vi "Autonomous Independent.vi"   [LabVIEW 2016]
doc: "This VI is called when autonomous begins, and will automatically be terminated when autonomous ends. You can carry out timed or sensor driven robot movement independently without needing to return to the caller."
uses:
  <vilib>/Rock Robotics/WPI/SafetyOutput/WPI_SafetyOutputConfigMenu.ctl
  <vilib>/Rock Robotics/WPI/Utilities/WPI_GetSetVariantRefNum.vi
  <vilib>/Rock Robotics/WPI/RobotDrive/WPI_RobotDriveArcadeDrive_Standard(NoSaturation).vi
panel:
  # "Be sure to right-click and choose Data Operations>>Make Current Value default if you want to save the array values with the VI"
types:
  T1 = typedef "WPI_SafetyOutputConfigMenu.ctl" = enum16{"Enable", "Disable"}
  T2 = typedef "WPI_JoystickDevRef.ctl" = cluster{"Device":T3}
  T3 = typedef "WPI_JoystickDeviceEnum.ctl" = enum16{"USB 0", "USB 1", "USB 2", "USB 3", "USB 4", "USB 5"}
  T4 = typedef "WPI_RobotDriveDevRef.ctl" = cluster{"DevStatus":errorcluster, "Motors[]":T5[], "Square Inputs":bool, "Max Output":dbl}
  T5 = typedef "WPI_MotorControlDeviceRef.ctl" = cluster{"DeviceStatus":errorcluster, "Type":T6, "PWM":cluster{"PWM Channel":T7, "DeadBand":T8}, "CAN":cluster{"Device Number":u8, "SetOutput VI Ref":variant, "GetOutput VI Ref":variant, "Enable VI Ref":variant, "Disable VI Ref":variant, "Data":variant}, "Invert":bool}
  T6 = typedef "WPI_MotorControlType.ctl" = enum16{"PWM", "CAN"}
  T7 = typedef "FPGA_DIOPWMChannel.ctl" = enum8{"PWM 0", "PWM 1", "PWM 2", "PWM 3", "PWM 4", "PWM 5", "PWM 6", "PWM 7", "PWM 8", "PWM 9", "PWM MXP 0", "PWM MXP 1", "PWM MXP 2", "PWM MXP 3", "PWM MXP 4", "PWM MXP 5", "PWM MXP 6", "PWM MXP 7", "PWM MXP 8", "PWM MXP 9", "Invalid"}
  T8 = typedef "WPI_PWMDeadband.ctl" = cluster{"Name":string, "maxPositivePwm":i32, "minPositivePwm":i32, "centerPwm":i32, "maxNegativePwm":i32, "minNegativePwm":i32, "angularRange":u16}
  T9 = cluster{"Buttons[0]":bool, "Buttons[1]":bool, "Buttons[2]":bool, "Buttons[3]":bool, "Buttons[4]":bool, "Buttons[5]":bool, "Buttons[6]":bool, "Buttons[7]":bool, "Buttons[8]":bool}
  T10 = cluster{"Yaw":dbl, "Roll":dbl, "Pitch":dbl, "Heading":dbl, "Fused Heading":dbl}
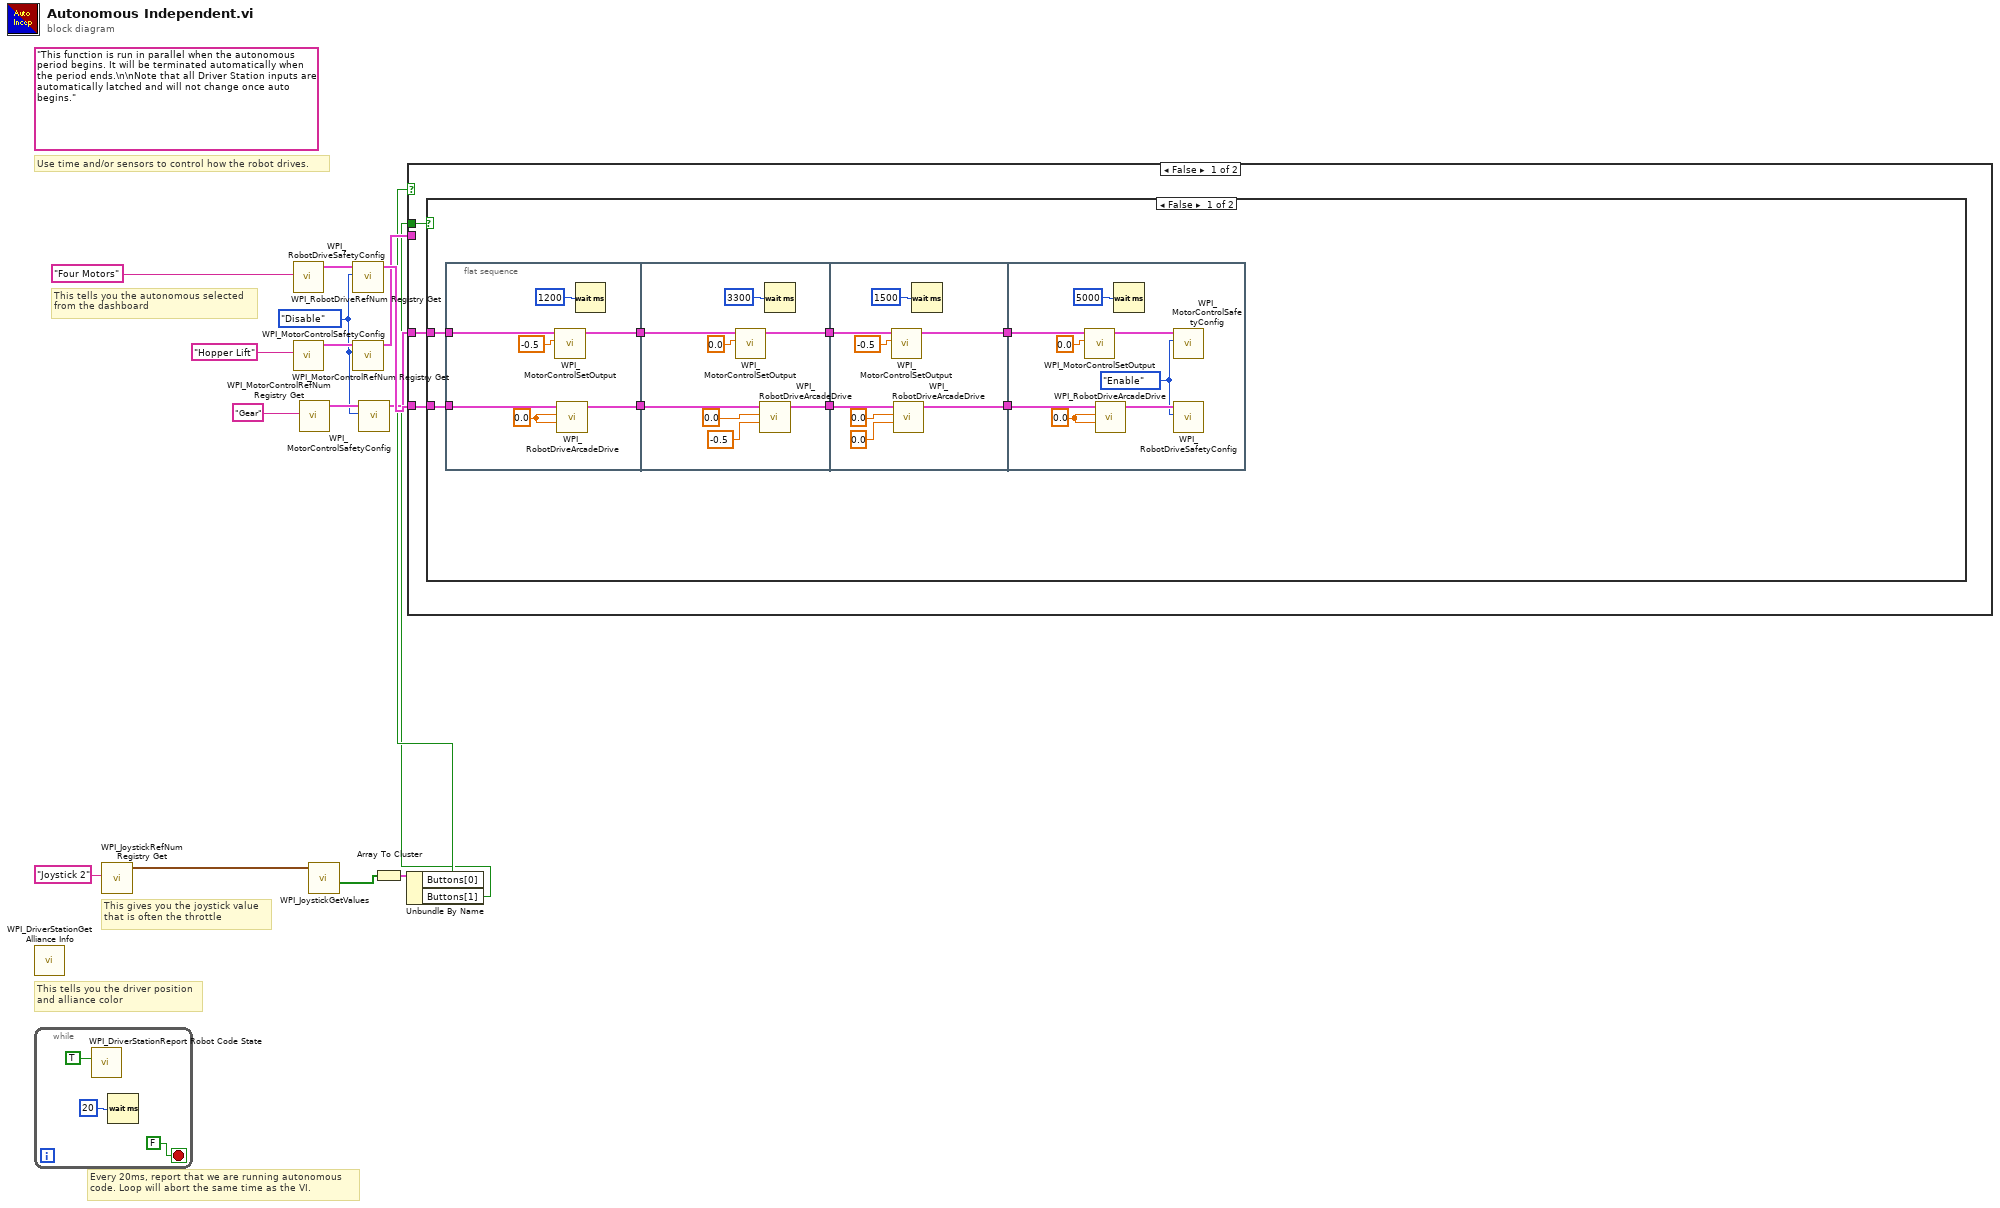
[diagram p0: block diagram]
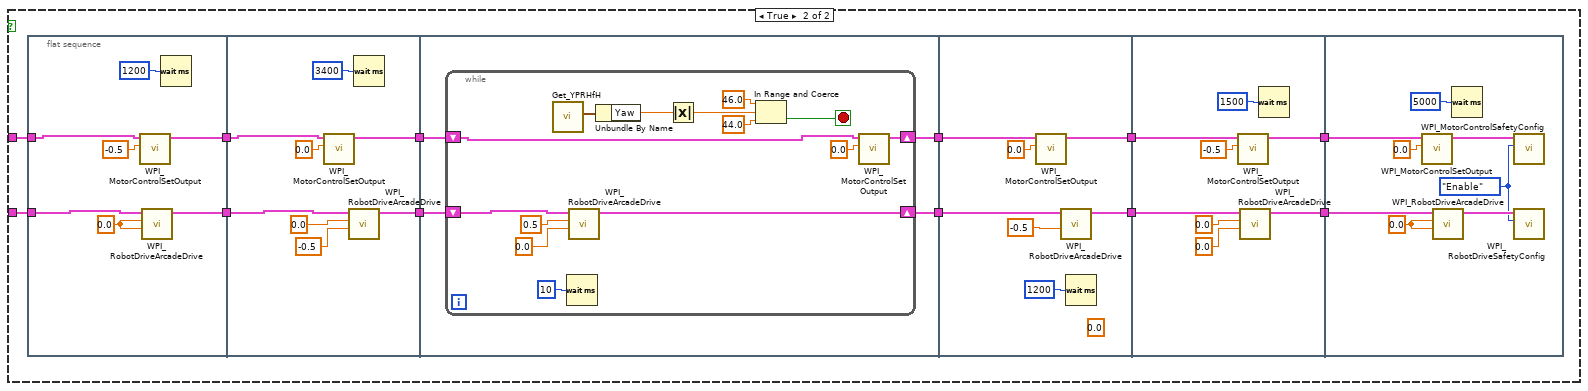
[diagram p2: hidden frame]
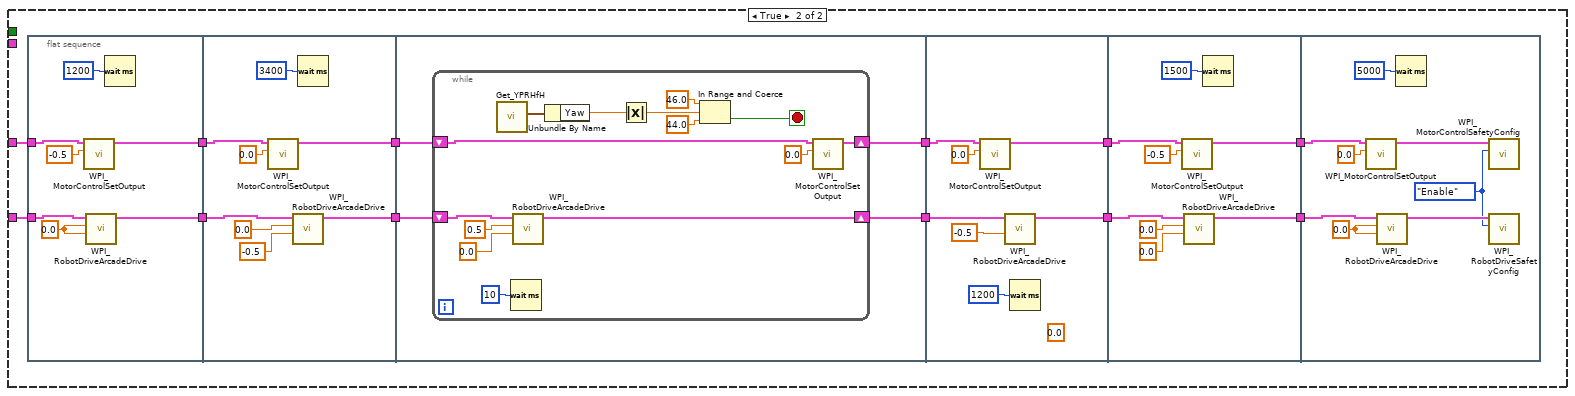
[diagram p3: hidden frame]
diagram:
  w6 = WPI_SafetyOutputConfigMenu."Disable" ("mode")
  (unwired) "This function is run in parallel when the autonomous period begins. It will be terminated automatically when the period ends.\n\nNote that all Driver Station inputs are automatically latched and will not change once auto begins."
  # "This tells you the autonomous selected\nfrom the dashboard"
  # "Every 20ms, report that we are running autonomous\ncode. Loop will abort the same time as the VI."
  # "This gives you the joystick value\nthat is often the throttle"
  # "Use time and/or sensors to control how the robot drives."
  # "This tells you the driver position\nand alliance color"
  n1 = call <vilib>:"WPI_DriverStationGet Alliance Info.vi"() -> ()  [unwired: 12 out]
  n2 = while {
    stop <- FALSE stop-if-true
    n3 = call <vilib>:"WPI_DriverStationReport Robot Code State.vi"("Autonomous"=TRUE) -> ()  [unwired: 10 in, 1 out]
    n4 = Wait (ms)(milliseconds to wait=u32 20) -> ()  [unwired: 1 out]
  }
  n5 = call <vilib>:"WPI_JoystickRefNum Registry Get.vi"("refnum name"="Joystick 2") -> ("JoystickDevRef"=w15:T2)  [unwired: 1 in, 9 out]
  n6 = call <vilib>:"WPI_RobotDriveRefNum Registry Get.vi"("refnum name"="Four Motors") -> ("RobotDriveDevRef"=w13:T4)  [unwired: 1 in, 9 out]
  n7 = call <vilib>:"WPI_MotorControlRefNum Registry Get.vi"("refnum name"="Hopper Lift") -> ("MotorControlDevRef"=w11:T5)  [unwired: 9 in, 1 out]
  n8 = call <vilib>:"WPI_MotorControlRefNum Registry Get.vi"("refnum name"="Gear") -> ("MotorControlDevRef"=w7:T5)  [unwired: 9 in, 1 out]
  n9 = call <vilib>:"WPI_JoystickGetValues.vi"("JoystickDevRef"=w15) -> ("Buttons"=w4:bool[])  [unwired: 6 in, 4 out]
  n10 = call <vilib>:"WPI_RobotDriveSafetyConfig.vi"("mode"=w6, "RobotDriveDevRef"=w13) -> ("RobotDriveDevRef"=w12:T4)  [unwired: 8 in, 1 out]
  n11 = call <vilib>:"WPI_MotorControlSafetyConfig.vi"("mode"=w6, "MotorControlDevRef"=w11) -> ("MotorControlDevRef"=w9:T5)  [unwired: 8 in, 1 out]
  n12 = call <vilib>:"WPI_MotorControlSafetyConfig.vi"("mode"=w6, "MotorControlDevRef"=w7) -> ("MotorControlDevRef"=w5:T5)  [unwired: 8 in, 1 out]
  n13 = Array To Cluster(array=w4) -> (cluster=w1:T9)
  n14 = Unbundle By Name(w1) -> ("Buttons[0]"=w3:bool, "Buttons[1]"=w2:bool)
  n15 = case shown="False" w3 {
    tunnel: w12 -> [w22 w130]
    tunnel: w9 -> [_ _]
    tunnel: w5 -> [w21 w131]
    tunnel: w2 -> [w20 _]
    frame False {
      n16 = case shown="False" w20 {
        tunnel: w22 -> [w28 w69]
        tunnel: w21 -> [w27 w68]
        frame False {
          n17 = flat-sequence {
            tunnel: w28 -> [w37]
            tunnel: [w36] -> w30
            tunnel: w27 -> [w34]
            tunnel: [w33] -> w29
            tunnel: w30 -> [w45]
            tunnel: [w44] -> w26
            tunnel: [w43] -> w24
            tunnel: w29 -> [w42]
            tunnel: w26 -> [w49]
            tunnel: [w48] -> w25
            tunnel: w24 -> [w47]
            tunnel: [w46] -> w23
            tunnel: w25 -> [w61]
            tunnel: w23 -> [w58]
            frame #0 {
              w35 = 0.0 ("X axis value")
              n18 = call <vilib>:"WPI_MotorControlSetOutput.vi"("Output"=-0.5, "MotorControlDevRef"=w34) -> ("MotorControlDevRef"=w33:T5)  [unwired: 7 in, 2 out]
              n19 = call-poly <vilib>:"WPI_RobotDriveArcadeDrive.vi"("Y axis value"=w35, "X axis value"=w35, "RobotDriveDevRef"=w37) -> ("RobotDriveDevRef"=w36:T4)  [unwired: 6 in, 2 out]
              n20 = Wait (ms)(milliseconds to wait=u32 1200) -> ()  [unwired: 1 out]
            }
            frame #1 {
              n21 = call <vilib>:"WPI_MotorControlSetOutput.vi"("Output"=0.0, "MotorControlDevRef"=w42) -> ("MotorControlDevRef"=w43:T5)  [unwired: 7 in, 2 out]
              n22 = call-poly <vilib>:"WPI_RobotDriveArcadeDrive.vi"("Y axis value"=-0.5, "X axis value"=0.0, "RobotDriveDevRef"=w45) -> ("RobotDriveDevRef"=w44:T4)  [unwired: 6 in, 2 out]
              n23 = Wait (ms)(milliseconds to wait=u32 3300) -> ()  [unwired: 1 out]
            }
            frame #2 {
              n24 = call <vilib>:"WPI_MotorControlSetOutput.vi"("Output"=-0.5, "MotorControlDevRef"=w47) -> ("MotorControlDevRef"=w46:T5)  [unwired: 7 in, 2 out]
              n25 = call-poly <vilib>:"WPI_RobotDriveArcadeDrive.vi"("Y axis value"=0.0, "X axis value"=0.0, "RobotDriveDevRef"=w49) -> ("RobotDriveDevRef"=w48:T4)  [unwired: 6 in, 2 out]
              n26 = Wait (ms)(milliseconds to wait=u32 1500) -> ()  [unwired: 1 out]
            }
            frame #3 {
              w59 = 0.0 ("Y axis value")
              w56 = WPI_SafetyOutputConfigMenu."Enable" ("mode")
              n27 = call <vilib>:"WPI_MotorControlSetOutput.vi"("Output"=0.0, "MotorControlDevRef"=w58) -> ("MotorControlDevRef"=w57:T5)  [unwired: 7 in, 2 out]
              n28 = call-poly <vilib>:"WPI_RobotDriveArcadeDrive.vi"("Y axis value"=w59, "X axis value"=w59, "RobotDriveDevRef"=w61) -> ("RobotDriveDevRef"=w60:T4)  [unwired: 6 in, 2 out]
              n29 = Wait (ms)(milliseconds to wait=u32 5000) -> ()  [unwired: 1 out]
              n30 = call <vilib>:"WPI_MotorControlSafetyConfig.vi"("mode"=w56, "MotorControlDevRef"=w57) -> ()  [unwired: 8 in, 2 out]
              n31 = call <vilib>:"WPI_RobotDriveSafetyConfig.vi"("mode"=w56, "RobotDriveDevRef"=w60) -> ()  [unwired: 8 in, 2 out]
            }
          }
        }
        frame True {
          n32 = flat-sequence {
            tunnel: w69 -> [w80]
            tunnel: [w79] -> w73
            tunnel: w68 -> [w77]
            tunnel: [w76] -> w72
            tunnel: w73 -> [w88]
            tunnel: [w87] -> w67
            tunnel: [w86] -> w66
            tunnel: w72 -> [w85]
            tunnel: w67 -> [w90]
            tunnel: w66 -> [w91]
            tunnel: [w89] -> w64
            tunnel: [w92] -> w63
            tunnel: [w110] -> w65
            tunnel: w64 -> [w108]
            tunnel: w63 -> [w111]
            tunnel: [w107] -> w62
            tunnel: [w117] -> w71
            tunnel: w65 -> [w116]
            tunnel: [w115] -> w70
            tunnel: w62 -> [w114]
            tunnel: w71 -> [w129]
            tunnel: w70 -> [w126]
            frame #0 {
              w78 = 0.0 ("X axis value")
              n33 = call <vilib>:"WPI_MotorControlSetOutput.vi"("Output"=-0.5, "MotorControlDevRef"=w77) -> ("MotorControlDevRef"=w76:T5)  [unwired: 7 in, 2 out]
              n34 = call-poly <vilib>:"WPI_RobotDriveArcadeDrive.vi"("Y axis value"=w78, "X axis value"=w78, "RobotDriveDevRef"=w80) -> ("RobotDriveDevRef"=w79:T4)  [unwired: 6 in, 2 out]
              n35 = Wait (ms)(milliseconds to wait=u32 1200) -> ()  [unwired: 1 out]
            }
            frame #1 {
              n36 = call <vilib>:"WPI_MotorControlSetOutput.vi"("Output"=0.0, "MotorControlDevRef"=w85) -> ("MotorControlDevRef"=w86:T5)  [unwired: 7 in, 2 out]
              n37 = call-poly <vilib>:"WPI_RobotDriveArcadeDrive.vi"("Y axis value"=-0.5, "X axis value"=0.0, "RobotDriveDevRef"=w88) -> ("RobotDriveDevRef"=w87:T4)  [unwired: 6 in, 2 out]
              n38 = Wait (ms)(milliseconds to wait=u32 3400) -> ()  [unwired: 1 out]
            }
            frame #2 {
              n39 = while {
                shift-right: [w101] -> w92
                shift-left: w91 -> [w104]
                shift-right: [w102] -> w89
                shift-left: w90 -> [w103]
                stop <- w99 stop-if-true
                n40 = call <vilib>:"Get_YPRHfH.vi"() -> ("YRPHfH"=w96:T10)  [unwired: 11 in]
                n41 = Wait (ms)(milliseconds to wait=u32 10) -> ()  [unwired: 1 out]
                n42 = call-poly <vilib>:"WPI_RobotDriveArcadeDrive.vi"("Y axis value"=0.0 ("X axis value"), "X axis value"=0.5 ("Y axis value"), "RobotDriveDevRef"=w103) -> ("RobotDriveDevRef"=w102:T4)  [unwired: 6 in, 2 out]
                n43 = Unbundle By Name(w96) -> ("Yaw"=w95:dbl)
                n44 = Absolute Value(x=w95) -> (abs(x)=w94:dbl)
                n45 = In Range and Coerce(upper limit=46.0, x=w94, lower limit=44.0) -> (In Range?=w99:bool)  [unwired: 1 out]
                n46 = call <vilib>:"WPI_MotorControlSetOutput.vi"("Output"=0.0, "MotorControlDevRef"=w104) -> ("MotorControlDevRef"=w101:T5)  [unwired: 7 in, 2 out]
              }
            }
            frame #3 {
              (unwired) 0.0 ("X axis value")
              n47 = call <vilib>:"WPI_MotorControlSetOutput.vi"("Output"=0.0, "MotorControlDevRef"=w111) -> ("MotorControlDevRef"=w110:T5)  [unwired: 7 in, 2 out]
              n48 = call-poly <vilib>:"WPI_RobotDriveArcadeDrive.vi"("Y axis value"=-0.5, "RobotDriveDevRef"=w108) -> ("RobotDriveDevRef"=w107:T4)  [unwired: 7 in, 2 out]
              n49 = Wait (ms)(milliseconds to wait=u32 1200) -> ()  [unwired: 1 out]
            }
            frame #4 {
              n50 = call <vilib>:"WPI_MotorControlSetOutput.vi"("Output"=-0.5, "MotorControlDevRef"=w116) -> ("MotorControlDevRef"=w115:T5)  [unwired: 7 in, 2 out]
              n51 = call-poly <vilib>:"WPI_RobotDriveArcadeDrive.vi"("Y axis value"=0.0, "X axis value"=0.0, "RobotDriveDevRef"=w114) -> ("RobotDriveDevRef"=w117:T4)  [unwired: 6 in, 2 out]
              n52 = Wait (ms)(milliseconds to wait=u32 1500) -> ()  [unwired: 1 out]
            }
            frame #5 {
              w127 = 0.0 ("Y axis value")
              w124 = WPI_SafetyOutputConfigMenu."Enable" ("mode")
              n53 = call <vilib>:"WPI_MotorControlSetOutput.vi"("Output"=0.0, "MotorControlDevRef"=w126) -> ("MotorControlDevRef"=w125:T5)  [unwired: 7 in, 2 out]
              n54 = call-poly <vilib>:"WPI_RobotDriveArcadeDrive.vi"("Y axis value"=w127, "X axis value"=w127, "RobotDriveDevRef"=w129) -> ("RobotDriveDevRef"=w128:T4)  [unwired: 6 in, 2 out]
              n55 = Wait (ms)(milliseconds to wait=u32 5000) -> ()  [unwired: 1 out]
              n56 = call <vilib>:"WPI_MotorControlSafetyConfig.vi"("mode"=w124, "MotorControlDevRef"=w125) -> ()  [unwired: 8 in, 2 out]
              n57 = call <vilib>:"WPI_RobotDriveSafetyConfig.vi"("mode"=w124, "RobotDriveDevRef"=w128) -> ()  [unwired: 8 in, 2 out]
            }
          }
        }
      }
    }
    frame True {
      n58 = flat-sequence {
        tunnel: w130 -> [w148]
        tunnel: [w147] -> w141
        tunnel: w131 -> [w145]
        tunnel: [w144] -> w140
        tunnel: w141 -> [w156]
        tunnel: [w155] -> w139
        tunnel: [w154] -> w138
        tunnel: w140 -> [w153]
        tunnel: w139 -> [w159]
        tunnel: w138 -> [w160]
        tunnel: [w158] -> w137
        tunnel: [w157] -> w136
        tunnel: [w178] -> w135
        tunnel: w137 -> [w176]
        tunnel: w136 -> [w179]
        tunnel: [w175] -> w134
        tunnel: [w185] -> w133
        tunnel: w135 -> [w184]
        tunnel: [w183] -> w132
        tunnel: w134 -> [w182]
        tunnel: w133 -> [w197]
        tunnel: w132 -> [w194]
        frame #0 {
          w146 = 0.0 ("X axis value")
          n59 = call <vilib>:"WPI_MotorControlSetOutput.vi"("Output"=-0.5, "MotorControlDevRef"=w145) -> ("MotorControlDevRef"=w144:T5)  [unwired: 7 in, 2 out]
          n60 = call-poly <vilib>:"WPI_RobotDriveArcadeDrive.vi"("Y axis value"=w146, "X axis value"=w146, "RobotDriveDevRef"=w148) -> ("RobotDriveDevRef"=w147:T4)  [unwired: 6 in, 2 out]
          n61 = Wait (ms)(milliseconds to wait=u32 1200) -> ()  [unwired: 1 out]
        }
        frame #1 {
          n62 = call <vilib>:"WPI_MotorControlSetOutput.vi"("Output"=0.0, "MotorControlDevRef"=w153) -> ("MotorControlDevRef"=w154:T5)  [unwired: 7 in, 2 out]
          n63 = call-poly <vilib>:"WPI_RobotDriveArcadeDrive.vi"("Y axis value"=-0.5, "X axis value"=0.0, "RobotDriveDevRef"=w156) -> ("RobotDriveDevRef"=w155:T4)  [unwired: 6 in, 2 out]
          n64 = Wait (ms)(milliseconds to wait=u32 3400) -> ()  [unwired: 1 out]
        }
        frame #2 {
          n65 = while {
            shift-right: [w169] -> w157
            shift-left: w160 -> [w172]
            shift-right: [w170] -> w158
            shift-left: w159 -> [w171]
            stop <- w167 stop-if-true
            n66 = call <vilib>:"Get_YPRHfH.vi"() -> ("YRPHfH"=w164:T10)  [unwired: 11 in]
            n67 = Wait (ms)(milliseconds to wait=u32 10) -> ()  [unwired: 1 out]
            n68 = call-poly <vilib>:"WPI_RobotDriveArcadeDrive.vi"("Y axis value"=0.0 ("X axis value"), "X axis value"=0.5 ("Y axis value"), "RobotDriveDevRef"=w171) -> ("RobotDriveDevRef"=w170:T4)  [unwired: 6 in, 2 out]
            n69 = Unbundle By Name(w164) -> ("Yaw"=w163:dbl)
            n70 = Absolute Value(x=w163) -> (abs(x)=w162:dbl)
            n71 = In Range and Coerce(upper limit=46.0, x=w162, lower limit=44.0) -> (In Range?=w167:bool)  [unwired: 1 out]
            n72 = call <vilib>:"WPI_MotorControlSetOutput.vi"("Output"=0.0, "MotorControlDevRef"=w172) -> ("MotorControlDevRef"=w169:T5)  [unwired: 7 in, 2 out]
          }
        }
        frame #3 {
          (unwired) 0.0 ("X axis value")
          n73 = call <vilib>:"WPI_MotorControlSetOutput.vi"("Output"=0.0, "MotorControlDevRef"=w179) -> ("MotorControlDevRef"=w178:T5)  [unwired: 7 in, 2 out]
          n74 = call-poly <vilib>:"WPI_RobotDriveArcadeDrive.vi"("Y axis value"=-0.5, "RobotDriveDevRef"=w176) -> ("RobotDriveDevRef"=w175:T4)  [unwired: 7 in, 2 out]
          n75 = Wait (ms)(milliseconds to wait=u32 1200) -> ()  [unwired: 1 out]
        }
        frame #4 {
          n76 = call <vilib>:"WPI_MotorControlSetOutput.vi"("Output"=-0.5, "MotorControlDevRef"=w184) -> ("MotorControlDevRef"=w183:T5)  [unwired: 7 in, 2 out]
          n77 = call-poly <vilib>:"WPI_RobotDriveArcadeDrive.vi"("Y axis value"=0.0, "X axis value"=0.0, "RobotDriveDevRef"=w182) -> ("RobotDriveDevRef"=w185:T4)  [unwired: 6 in, 2 out]
          n78 = Wait (ms)(milliseconds to wait=u32 1500) -> ()  [unwired: 1 out]
        }
        frame #5 {
          w195 = 0.0 ("Y axis value")
          w192 = WPI_SafetyOutputConfigMenu."Enable" ("mode")
          n79 = call <vilib>:"WPI_MotorControlSetOutput.vi"("Output"=0.0, "MotorControlDevRef"=w194) -> ("MotorControlDevRef"=w193:T5)  [unwired: 7 in, 2 out]
          n80 = call-poly <vilib>:"WPI_RobotDriveArcadeDrive.vi"("Y axis value"=w195, "X axis value"=w195, "RobotDriveDevRef"=w197) -> ("RobotDriveDevRef"=w196:T4)  [unwired: 6 in, 2 out]
          n81 = Wait (ms)(milliseconds to wait=u32 5000) -> ()  [unwired: 1 out]
          n82 = call <vilib>:"WPI_MotorControlSafetyConfig.vi"("mode"=w192, "MotorControlDevRef"=w193) -> ()  [unwired: 8 in, 2 out]
          n83 = call <vilib>:"WPI_RobotDriveSafetyConfig.vi"("mode"=w192, "RobotDriveDevRef"=w196) -> ()  [unwired: 8 in, 2 out]
        }
      }
    }
  }
